vi "Write dt.vi"(8 "error in (no error)":errorcluster, 10 "dt":dbl=1.0, 11 "PID Control in":refnum<class "PID Control.lvclass">) -> (0 "error out":errorcluster, 3 "PID Control out":refnum<class "PID Control.lvclass">)   [LabVIEW 2016, in "PID Control.lvclass"]
uses:
  PID Control.lvclass
  PID Control.lvclass/PID Control.ctl
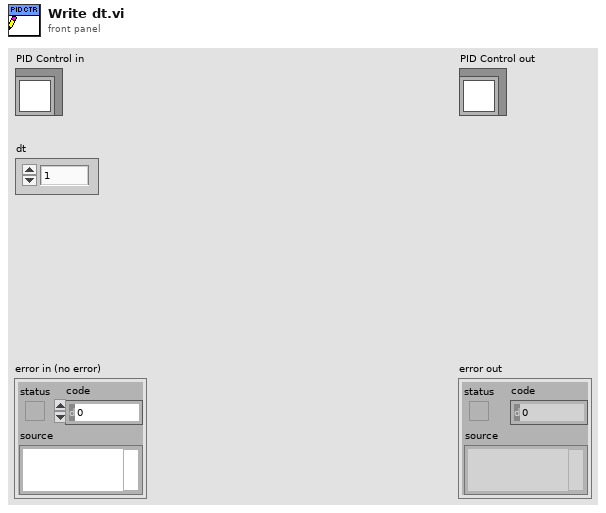
[diagram p1: front panel]
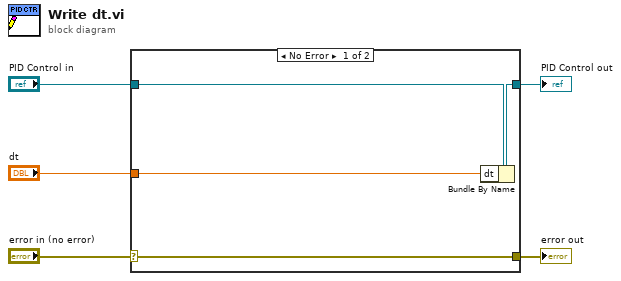
[diagram p0: block diagram]
diagram:
  n1 = case shown="No Error" "error in (no error)" {
    selector: "error in (no error)" -> [w9 w10]
    tunnel: [w9 w10] -> w4
    tunnel: [w7 w11] -> w2
    tunnel: "PID Control in" -> [w8 w11]
    tunnel: "dt" -> [w6 _]
    frame No Error {
      n2 = Bundle By Name(cluster=w8, "dt"=w6) -> (w7:refnum<class "PID Control.lvclass">)
    }
    frame Error {
    }
  }
  "error out" <- w4
  "PID Control out" <- w2
